vi "MT QAM Align to Ideal Symbols.vi"() -> (15 "Error Out":errorcluster)   [LabVIEW 2010]
doc: "This example demonstrates the symbol alignment in a QAM Modulation Demodulation system."
uses:
  <vilib>/AddOns/Modulation/Digital/General/MT Generate QAM System Parameters(M).vi
  <vilib>/addons/Modulation/Digital/General/MT Generate Bits (Galois, PN Order).vi
  <vilib>/AddOns/Modulation/Digital/General/MT Map Bits to QAM Symbols.vi
  <vilib>/AddOns/Modulation/Digital/General/MT Apply Pulse Shaping Filter (Generic).vi
  <vilib>/AddOns/Modulation/Digital/General/MT Apply Matched Filter (Generic).vi
  <vilib>/AddOns/Modulation/Digital/General/MT Map QAM Symbols to Bits.vi
  <vilib>/AddOns/Modulation/Digital/Demodulation/MT Calculate BER After Trigger (PN Sequence).vi
  <vilib>/AddOns/Modulation/Digital/General/MT Align to Ideal Symbols (Generic).vi
  <vilib>/addons/Modulation/niDMT.lvlib
  <vilib>/addons/Modulation/niAMT.lvlib
panel:
  in  "Align to Ideal Symbols ? (T)":bool=TRUE
  out "Bit Error Rate":dbl format="%.4f"
  in  "PN Sequence Order (9)":i32=9
  in  "M-QAM Symbols":i32=10000
  in  "M-QAM":i32=256
  in  "Samples per Symbol":i32=4
  in  "Pulse Shaping Filter":T1(ring)=enum."Root Raised Cos"
  in  "Maximum Symbol Timing Ambiguity":dbl=5.0
  in  "autoscale":bool
  out "Symbol Timing Ambiguity (symbols)":dbl=2.1334297225143106
  out "Constellation Graph Post Demodulation":T2(graph)
  # "NOTE:\nRun this example in continuous mode to see the effect of \"Align to Ideal Symbols\" boolean control"
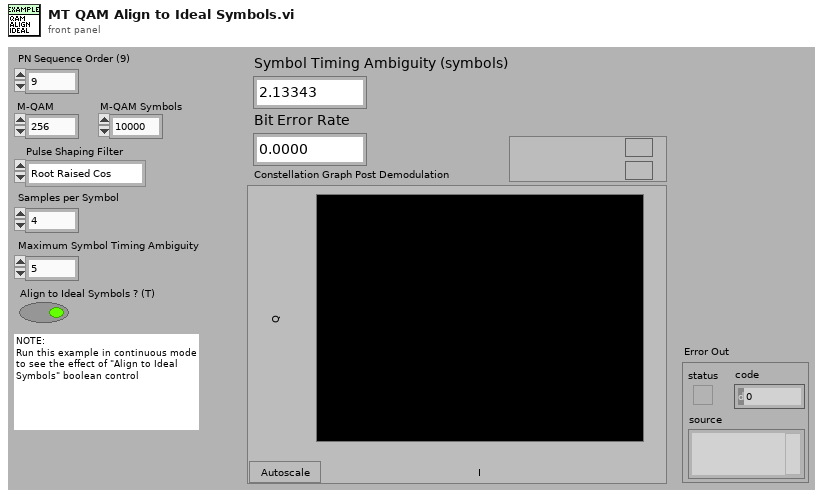
[diagram p1: front panel]
types:
  T1 = enum16{"none", "Raised Cosine", "Root Raised Cos", "Gaussian"}
  T2 = cluster{"Decimated Array":dbl[], "Decimated Array":dbl[]}[]
  T3 = cluster{"samples per symbol (16)":i32, "symbol map":cdb[]}
  T4 = typedef "niAMT.lvlib/Complex Data Waveform.ctl" = cluster{"t0":dbl, "dt":dbl, "Y":cdb[]}
  T5 = cluster{"constellation":dbl[], "oversampled data":dbl[]}[]
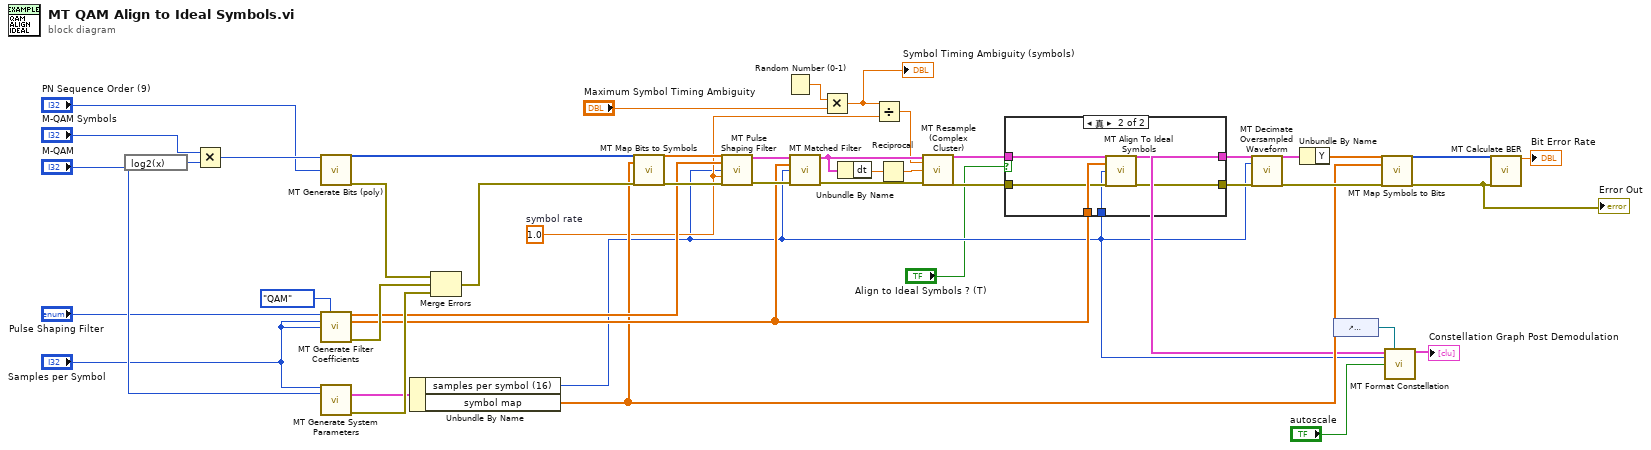
[diagram p0: block diagram]
diagram:
  w12 = 1.0  # symbol rate
  n1 = expression code="log2(x)"("M-QAM") -> (w7:i32)
  n2 = Multiply(x="M-QAM Symbols", y=w7) -> (x*y=w42:i32)
  n3 = call-poly <vilib>:"MT Generate Bits (poly).vi"("total bits (128)"=w42, "PN sequence order (9)"="PN Sequence Order (9)") -> ("output bit stream"=w40:i8[], "error out"=w39:errorcluster)  [unwired: 3 in, 9 out]
  n4 = call <vilib>:"MT Generate Filter Coefficients.vi"("pulse shaping filter (none)"="Pulse Shaping Filter", "modulation type"=enum16{"FSK", "PSK", "QAM", "MSK", "PAM", "ASK"}."QAM", "pulse shaping samples per symbol (16)"="Samples per Symbol", "matched samples per symbol (16)"="Samples per Symbol") -> ("pulse shaping filter coefficients"=w33:dbl[], "matched filter coefficients"=w28:dbl[], "error out"=w38:errorcluster)  [unwired: 3 in, 6 out]
  n5 = call-poly <vilib>:"MT Generate System Parameters.vi"("samples per symbol (16)"="Samples per Symbol", "M-QAM (16)"="M-QAM") -> ("QAM system parameters"=w27:T3, "error out"=w37:errorcluster)  [unwired: 3 in, 9 out]
  n6 = Unbundle By Name(w27) -> ("samples per symbol (16)"=w9:i32, "symbol map"=w24:cdb[])
  n7 = Merge Errors(w39, w38, w37) -> (w36:errorcluster)
  n8 = call-poly <vilib>:"MT Map Bits to Symbols.vi"("input bit stream"=w40, "symbol map"=w24, "error in (no error)"=w36) -> ("symbols"=w34:cdb[], "error out"=w35:errorcluster)  [unwired: 1 in, 10 out]
  n9 = call-poly <vilib>:"MT Pulse Shaping Filter.vi"("symbols"=w34, "pulse shaping filter coefficients"=w33, "samples per symbol (16)"=w9, "symbol rate (Hz)"=w12, "error in (no error)"=w35) -> ("output complex waveform"=w32:T4, "error out"=w31:errorcluster)  [unwired: 1 in, 8 out]
  n10 = Random Number (0-1)() -> (number: 0 to 1=w17:dbl)
  n11 = call-poly <vilib>:"MT Matched Filter.vi"("input complex waveform"=w32, "matched filter coefficients"=w28, "samples per symbol (16)"=w9, "error in (no error)"=w31) -> ("output complex waveform"=w20:T4, "error out"=w30:errorcluster)  [unwired: 1 in, 9 out]
  n12 = Multiply(x=w17, y="Maximum Symbol Timing Ambiguity") -> (x*y=w10:dbl)
  "Symbol Timing Ambiguity (symbols)" <- w10
  n13 = Unbundle By Name(w20) -> ("dt"=w19:dbl)
  n14 = Divide(x=w10, y=w12) -> (x/y=w11:dbl)
  n15 = Reciprocal(x=w19) -> (1/x=w18:dbl)
  n16 = call <vilib>:"MT Resample (Complex Cluster).vi"("input complex waveform"=w20, "initial sample offset (sec)"=w11, "desired sample rate (Hz)"=w18, "error in (no error)"=w30) -> ("output complex waveform"=w21:T4, "error out"=w22:errorcluster)  [unwired: 2 in, 8 out]
  n17 = case shown="真" "Align to Ideal Symbols ? (T)" {
    tunnel: [w46 w53] -> w29
    tunnel: w28 -> [_ w52]
    tunnel: w22 -> [w46 w51]
    tunnel: w21 -> [w47 w50]
    tunnel: [w47 w49] -> w13
    tunnel: w9 -> [_ w48]
    frame False {
    }
    frame True {
      n18 = call-poly <vilib>:"MT Align To Ideal Symbols.vi"("input complex waveform"=w50, "matched filter coefficients"=w52, "samples per symbol (16)"=w48, "error in (no error)"=w51) -> ("output complex waveform"=w49:T4, "error out"=w53:errorcluster)  [unwired: 1 in, 9 out]
    }
  }
  n19 = call <vilib>:"MT Decimate Oversampled Waveform.vi"("input complex waveform"=w13, "decimation factor"=w9, "error in (no error)"=w29) -> ("output complex waveform"=w25:T4, "error out"=w26:errorcluster)  [unwired: 2 in, 9 out]
  n20 = Unbundle By Name(w25) -> ("Y"=w23:cdb[])
  n21 = control-ref of="Constellation Graph Post Demodulation"() -> (w14:refnum<vi>)
  n22 = call-poly <vilib>:"MT Map Symbols to Bits.vi"("symbols"=w23, "symbol map"=w24, "error in (no error)"=w26) -> ("output bit stream"=w44:i8[], "error out"=w45:errorcluster)  [unwired: 11 out]
  "Error Out" <- w45
  n23 = call <vilib>:"MT Format Constellation.vi"("waveform"=w13, "constellation reference"=w14, "samples per symbol"=w9, "autoscale"="autoscale") -> ("constellation graph"=→"Constellation Graph Post Demodulation":T5)  [unwired: 1 in, 10 out]
  n24 = call-poly <vilib>:"MT Calculate BER.vi"("input bit stream"=w44, "error in (no error)"=w45) -> ("BER"=→"Bit Error Rate":dbl)  [unwired: 4 in, 9 out]
